vi "Creators Creator Queue Alias.vi"(11 "eeeee in":refnum<class "eeeee.lvclass">) -> (2 "Creator Queue Alias":string, 3 "eeeee out":refnum<class "eeeee.lvclass">)   [LabVIEW 2021, in "Providers.lvlib" / "eeeee.lvlib" / "eeeee.lvclass"]
uses:
  eeeee.lvclass
  eeeee.lvclass/eeeee.ctl
  jettl/Event/Event.lvclass
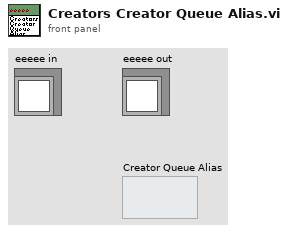
[diagram p1: front panel]
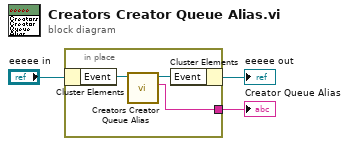
[diagram p0: block diagram]
diagram:
  n1 = in-place {
    in-place-border: [w4] -> w1
    n2 = in-place-cluster #1("eeeee in") -> ("Event"=w6:refnum<class "Event.lvclass">)
    n3 = call-dynamic "Creators Creator Queue Alias.vi"("Event in"=w6) -> ("Creator Queue Alias"=w4:string, "Event out"=w5:refnum<class "Event.lvclass">)  [unwired: 9 in]
    n4 = in-place-cluster #1("Event"=w5) -> (→"eeeee out":refnum<class "eeeee.lvclass">)
  }
  "Creator Queue Alias" <- w1
